vi "load data ver 2.vi"() -> ()   [LabVIEW 2016]
uses:
  Detect Threshold Control.ctl
  <vilib>/Utility/file.llb/Read Delimited Spreadsheet (DBL).vi
  <vilib>/ptbypt/NI_PtbyPt.lvlib
  <vilib>/Analysis/NI_AAL_SigProc.lvlib
  <vilib>/addons/Biomedical/NI_BMTK_Measurements.lvlib
panel:
  out "QRS peak":dbl[](array[numeric])
  out "QRS time":dbl[](array[numeric])
  out "BPM (output)":string
  out "Filter 2":dbl(graph)
  out "BPM":dbl
  in  "order":i32=4
  out "Filter":dbl[](graph)
  out "detected frequency":dbl format="%.2p"
  in  "stop":bool
  out "Data":dbl[](graph)=[0.3577, 0.3626, 0.3626, 0.3724, 0.3822, 0.4018, 0.4165, 0.441, 0.4557, 0.4753, 0.4704, 0.4704, 0.4704, 0.4557, 0.4312, 0.4214, 0.3969, 0.3724, 0.343, 0.3234, 0.3136, 0.3038, 0.3038, 0.3038, 0.2989, 0.3087, 0.3136, 0.3185, 0.3234, 0.3185, 0.3283, 0.3283, 0.3332, 0.3332, 0.3283, 0.3038, 0.2989, 0.3038, 0.3871, 0.5488, 0.784, 1.0094, 1.176, 1.1907, 1.078, 0.833, 0.5488, 0.2989, 0.1323, 0.0539, 0.0392, 0.0539, 0.0637, 0.0931, 0.1078, 0.1274, 0.1372, 0.1617, 0.1715, 0.1911, 0.2009, 0.2205, 0.2254, 0.2499, 0.2597, 0.2744, 0.2793, 0.294, 0.3038, 0.3185, 0.3234, 0.3332, 0.3479, 0.3528, 0.3528, 0.3577, 0.3626, 0.3724, 0.3822, 0.3871, 0.392, 0.4018, 0.4067, 0.4214, 0.4312, 0.4459, 0.4508, 0.4606, 0.4557, 0.4508, 0.4459, 0.4214, 0.4067, 0.3773, 0.3626, 0.3332, 0.3038, 0.2646, 0.245, 0.2205]
  out "dt":dbl=0.01
  out "DC estimate (V)":dbl format="%0.2f"
  out "Frequency":cluster{"f0":dbl, "df":dbl, "magnitude":dbl[]}(graph)={"f0"=0.0, "df"=1.0, "magnitude"=[0.0001493041908513748, 0.0011863720398903287, 0.0018747594052843446, 0.0006839329838492028, 0.00013714296027994926, 6.6574800709562e-05, 5.393826672564763e-06, 9.671137080398512e-07, 1.8688707585130385e-07, 3.0218494488076384e-08, 1.1119287573191355e-08, 2.5143270250361713e-08, 2.4194499002579346e-08, 2.1468803799325076e-08, 1.1286079164884523e-08, 5.722127749122396e-09, 2.674472525144362e-09, 1.0101846977742842e-09, 6.471424440126323e-10, 5.410401195181136e-10, 3.9516263871947605e-10, 2.8129643689443643e-10, 1.612108080759511e-10, 8.938815192316474e-11, 5.171141729498619e-11, 3.138614192720704e-11, 2.3523983292897458e-11, 1.5562261469458817e-11, 1.1127723227989894e-11, 7.1069770220219995e-12, 4.06402298369841e-12, 2.7950349836912914e-12, 1.5494858759679864e-12, 1.116974489135686e-12, 7.202482820748693e-13, 3.58622786094221e-13, 2.889039602992115e-13, 1.5942724470189004e-13, 1.0131664723341154e-13, 2.5170376802722627e-14, 1.1185496914759323e-14, 2.877485304016703e-14, 3.628167303865536e-15, 4.900590573038349e-15, 1.8904225729518165e-15, 1.603897058080336e-16, 5.022679134694723e-16, 4.657147849371043e-17, 1.1634890589264188e-16, 7.550759596510883e-17]}
  in  "Index data":i32=4
  in  "#samples read":u32=50
  in  "Fs":u32=200
  in  "file path (dialog if empty)":path=path "C:/Users/Le Thanh Nhan/Desktop/Arduino_datalogger/nhan140518140435.csv"
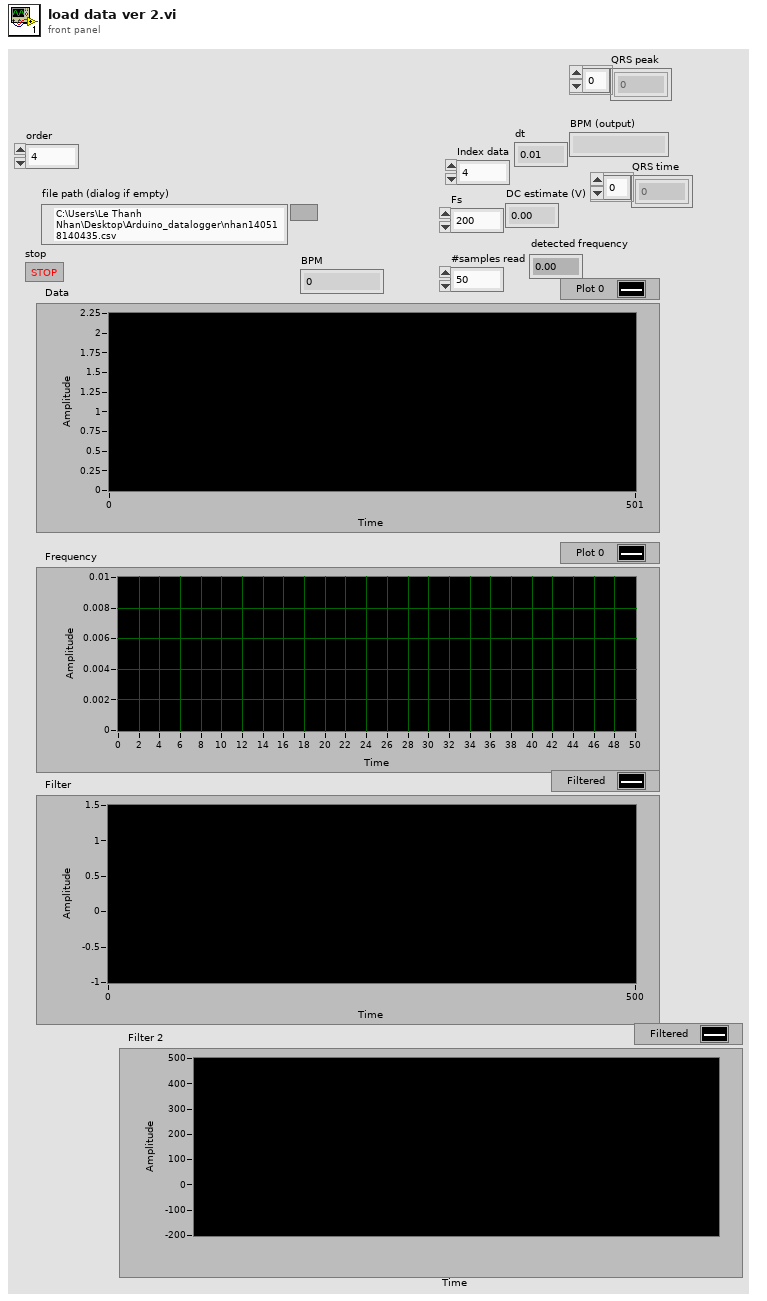
[diagram p1: front panel]
types:
  T1 = cluster{"peak detection initial threshold":dbl, "threshold factor":dbl}
  T2 = typedef "Detect Threshold Control.ctl" = enum16{"Get Threshold", "Pulse Found", "Pulse Not Found"}
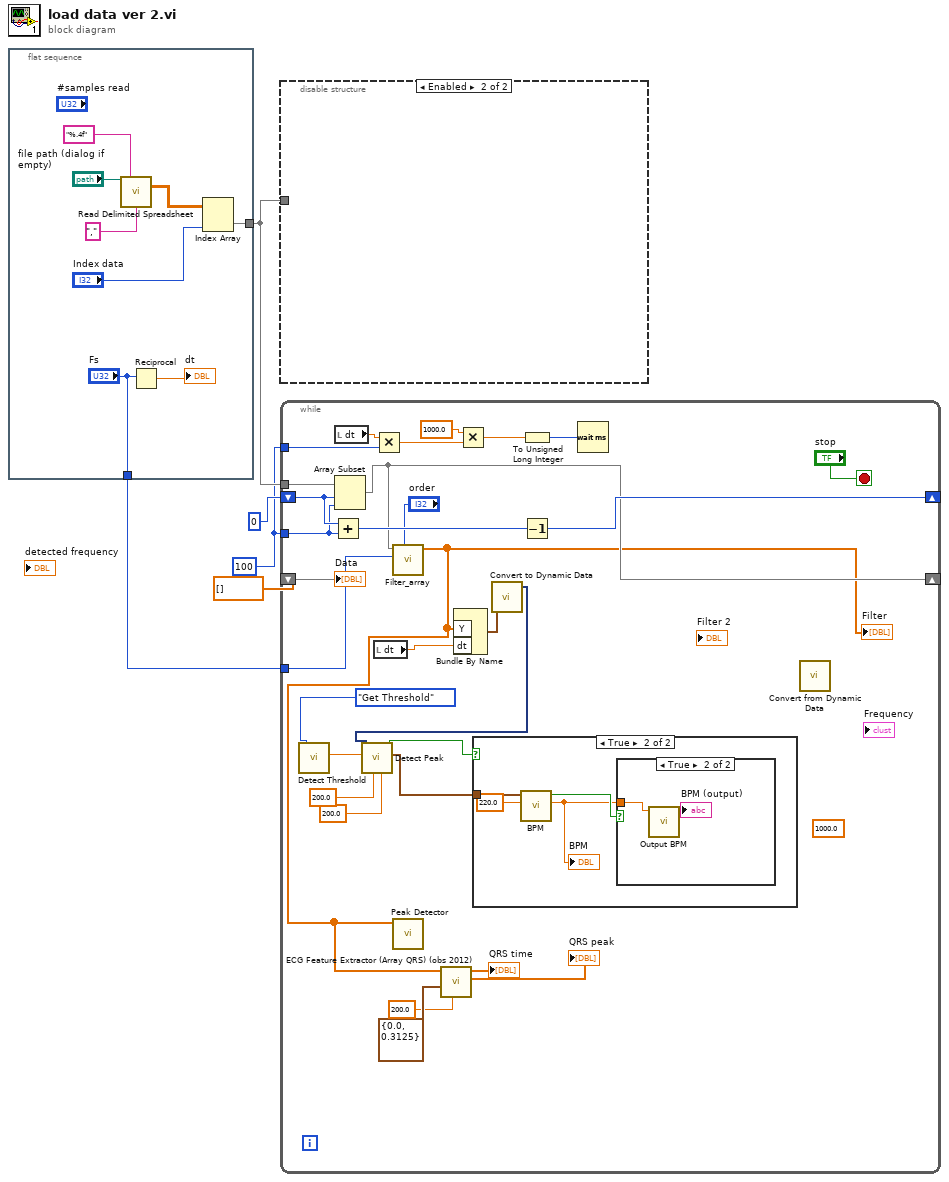
[diagram p0: block diagram]
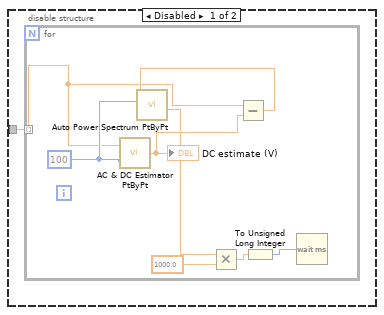
[diagram p2: hidden frame]
diagram:
  w3 = 100 ("length")
  n1 = flat-sequence {
    tunnel: [w8] -> w4
    tunnel: ["Fs"] -> w2
    frame #0 {
      n2 = call-poly <vilib>:"Read Delimited Spreadsheet.vi"("file path (dialog if empty)"="file path (dialog if empty)", "format (%.3f)"="%.4f", "delimiter (\\t)"="," ("delimiter (\\t)")) -> ("all rows"=w10:dbl[][])  [unwired: 7 in, 5 out]
      n3 = Reciprocal(x="Fs") -> (1/x=→"dt":dbl)
      n4 = Index Array(array=w10, index (col)="Index data") -> (element=w8:dbl[])  [unwired: 1 in]
    }
  }
  n5 = disable-structure shown="Enabled" {
    disable-tunnel: w4 -> [w14 _]
    frame Disabled {
      n6 = for {
        tunnel: w14 -> [w16] mode=indexing
        w19 = 100 ("sample length")
        n7 = call <vilib>:"AC & DC Estimator PtByPt.vi"("signal"=w16, "sample length"=w19) -> ("DC estimate (V)"=w18:dbl)  [unwired: 1 in, 2 out]
        "DC estimate (V)" <- w18
        n8 = Multiply(y=1000.0) -> (x=w15:dbl, x*y=w21:dbl)
        n9 = Subtract(x=w16, y=w18) -> (x-y=w17:dbl)
        n10 = call <vilib>:"Auto Power Spectrum PtByPt.vi"("signal"=w17, "sample length"=w19, "dt"=w15) -> ()  [unwired: 2 in, 3 out]
        n11 = To Unsigned Long Integer(number=w21) -> (unsigned 32bit integer=w20:u32)
        n12 = Wait (ms)(milliseconds to wait=w20) -> ()  [unwired: 1 out]
      }
    }
    frame Enabled {
    }
  }
  n13 = while {
    tunnel: w3 -> [w51]
    shift-right: [w49] -> _
    shift-left: 0 ("index") -> [w52]
    tunnel: w4 -> [w47]
    shift-right: [w28] -> _
    shift-left: dbl[] [] -> [w38]
    tunnel: w3 -> [w46]
    tunnel: w2 -> [w40]
    stop <- "stop" stop-if-true
    (unwired) 1000.0 ("y")
    n14 = call "Detect Threshold.vi"("Action"=Detect_Threshold_Control."Get Threshold") -> ("Threshold"=w36:dbl)  [unwired: 5 in, 1 out]
    n15 = Add(x=w52, y=w51) -> (x+y=w50:i32)
    n16 = local read "dt"() -> (w44:dbl)
    n17 = Array Subset(array=w47, index=w52, length=w51) -> (w28:dbl[])
    n18 = Multiply(x=w44, y=w46) -> (x*y=w43:dbl)
    n19 = local read "dt"() -> (w29:dbl)
    n20 = call "Filter_array.vi"("order"="order", "sampling freq: fs"=w40, "Input"=w28) -> ("Filtered"=w23:dbl[])  [unwired: 8 in]
    "Filter" <- w23
    n21 = call <vilib>:"Peak Detector.vi"("X"=w23) -> ()  [unwired: 6 in, 5 out]
    n22 = call <vilib>:"ECG Feature Extractor (Array QRS) (obs 2012).vi"("sampling rate"=200.0, "QRS detector parameters"=T1 {"peak detection initial threshold"=0.0, "threshold factor"=0.3125}, "ECG"=w23) -> ("QRS peak"=→"QRS peak":dbl[], "QRS time"=→"QRS time":dbl[])  [unwired: 6 in, 1 out]
    n23 = Bundle By Name("Y"=w23, "dt"=w29) -> (w31:waveform(dbl))  [unwired: 1 in]
    n24 = Multiply(x=1000.0 ("x*y"), y=w43) -> (x*y=w41:dbl)
    n25 = call "Convert to Dynamic Data"("Waveform"=w31) -> ("Dynamic Data Type"=w30:dynamicdata)  [unwired: 3 in]
    n26 = call "Detect Peak.vi"("Num Samples"=200.0, "Rate"=200.0, "Threshold"=w36, "Filtered Signal"=w30) -> ("Peak Time Stamp"=w34:timestamp, "Peak Found?"=w35:bool)  [unwired: 4 in, 2 out]
    n27 = case shown="True" w35 {
      tunnel: w34 -> [_ w56]
      frame False {
      }
      frame True {
        n28 = call "BPM.vi"("Max BPM Threshold"=220.0, "Time Stamp"=w56) -> ("BPM"=w53:dbl, "Below MAX BPM Threshold?"=w54:bool)  [unwired: 3 in, 1 out]
        "BPM" <- w53
        n29 = case shown="True" w54 {
          tunnel: w53 -> [_ w58]
          frame False {
          }
          frame True {
            n30 = call "Output BPM.vi"("BPM (input)"=w58) -> ("BPM (output)"=→"BPM (output)":string)  [unwired: 5 in, 1 out]
          }
        }
      }
    }
    n31 = To Unsigned Long Integer(number=w41) -> (unsigned 32bit integer=w45:u32)
    n32 = Decrement(x=w50) -> (x-1=w49:i32)
    n33 = Wait (ms)(milliseconds to wait=w45) -> ()  [unwired: 1 out]
    n34 = call "Convert from Dynamic Data"() -> ()  [unwired: 4 in, 1 out]
    "Data" <- w38
  }
